vi "+S2C_VLFT10_Process.vi"(8 "Error In":errorcluster) -> (0 "Error Out":errorcluster)   [LabVIEW 2015]
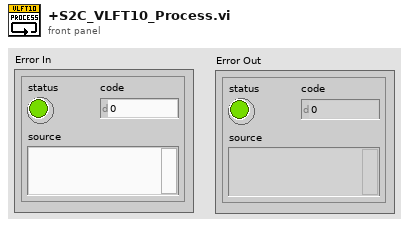
[diagram p1: front panel]
types:
  T1 = cluster{"Caller-Q":refnum<queue>, "Command":string, "Return":string, "Data":variant, "Timeout":dbl}
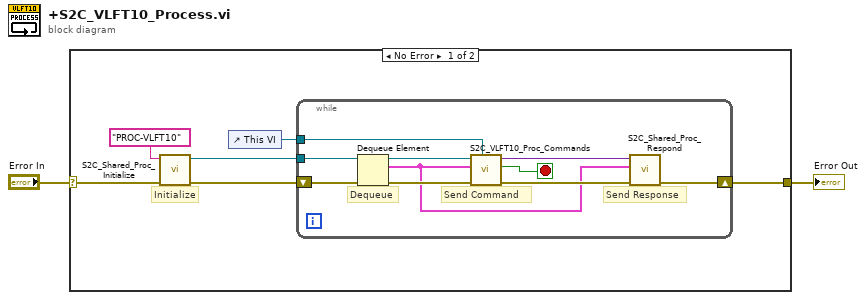
[diagram p0: block diagram]
diagram:
  n1 = case shown="No Error" "Error In" {
    selector: "Error In" -> [w7 w19]
    tunnel: [w8 w19] -> w1
    frame No Error {
      # "Initialize"
      n2 = call "S2C_Shared_Proc_Initialize.vi"("Error In"=w7, "Q-Name"="PROC-VLFT10" ("name (unnamed)")) -> ("Error Out"=w6:errorcluster, "Q-Ref"=w5:refnum<queue>)  [unwired: 8 in]
      n3 = control-ref of="This VI"() -> (w3:refnum<vi>)
      n4 = while {
        shift-right: [w16] -> w8
        shift-left: w6 -> [w18]
        tunnel: w5 -> [w17]
        tunnel: w3 -> [w9]
        stop <- w12 stop-if-true
        # "Send Command"
        # "Send Response"
        # "Dequeue"
        n5 = Dequeue Element(queue=w17, error in (no error)=w18) -> (queue out=w10:refnum<queue>, element=w11:T1, error out=w15:errorcluster)  [unwired: 1 in, 1 out]
        n6 = call "S2C_VLFT10_Proc_Commands.vi"("VI_Ref"=w9, "Error In"=w15, "Settings"=w11, "Q-Ref"=w10) -> ("Error Out"=w13:errorcluster, "Exit?"=w12:bool, "Response"=w14:variant)  [unwired: 5 in]
        n7 = call "S2C_Shared_Proc_Respond.vi"("Error In"=w13, "Settings"=w11, "Response"=w14) -> ("Error Out"=w16:errorcluster)  [unwired: 8 in]
      }
    }
    frame Error {
    }
  }
  "Error Out" <- w1
